vi "hw9p4_hickey.vi"() -> ()   [LabVIEW 2014]
panel:
  out "Prime?":bool
  in  "Integer":dbl
  # "101467 is not prime"
  # "102703 is not prime"
  # "97861 is prime"
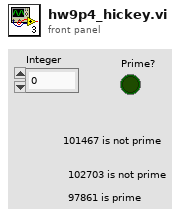
[diagram p1: front panel]
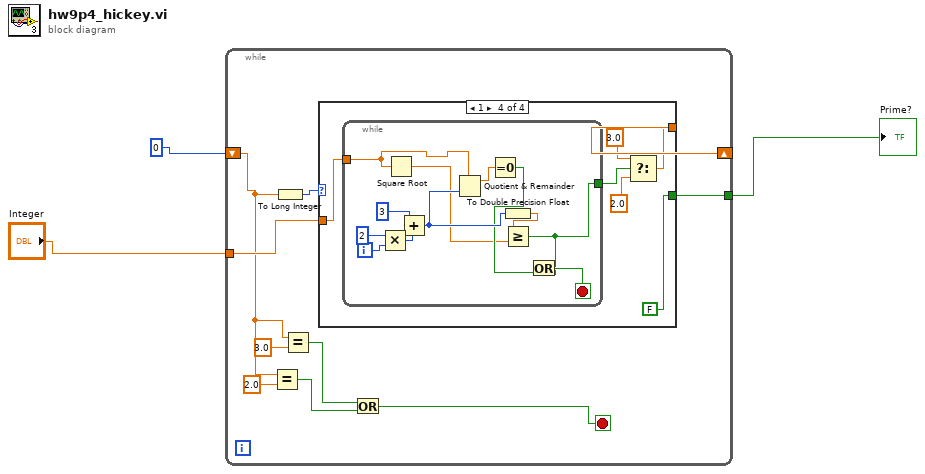
[diagram p0: block diagram]
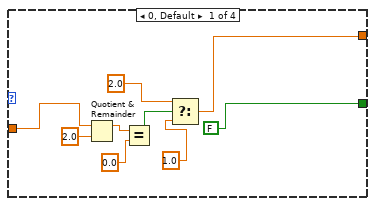
[diagram p2: hidden frame]
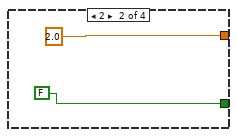
[diagram p3: hidden frame]
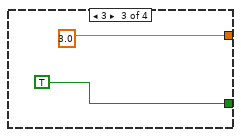
[diagram p4: hidden frame]
diagram:
  n1 = while {
    shift-right: [w12] -> _
    shift-left: 0 -> [w6]
    tunnel: "Integer" -> [w13]
    tunnel: [w4] -> w1
    stop <- w7 stop-if-true
    n2 = Equal?(x=w6, y=2.0) -> (x = y?=w10:bool)
    n3 = To Long Integer(number=w6) -> (32bit integer=w5:i32)
    n4 = Equal?(x=w6, y=3.0) -> (x = y?=w8:bool)
    n5 = case shown="1" w5 {
      tunnel: w13 -> [w21 _ _ w32]
      tunnel: [w15 2.0 ("y") 3.0 ("y") w28] -> w12
      tunnel: [FALSE FALSE TRUE FALSE] -> w4
      frame 0, Default {
        n6 = Quotient & Remainder(x=w21, y=2.0) -> (x-y*floor(x/y)=w19:dbl)  [unwired: 1 out]
        n7 = Equal?(x=w19, y=0.0 ("t")) -> (x = y?=w17:bool)
        n8 = Select(t=2.0, s=w17, f=1.0 ("t")) -> (s? t:f=w15:dbl)
      }
      frame 2 {
      }
      frame 3 {
      }
      frame 1 {
        n9 = while {
          tunnel: w32 -> [w38]
          tunnel: [w33] -> w27
          i -> [w44]
          stop <- w37 stop-if-true
          n10 = Multiply(x=2, y=w44) -> (x*y=w42:i32)
          n11 = Square Root(x=w38) -> (sqrt(x)=w35:dbl)
          n12 = Add(x=3, y=w42) -> (x+y=w39:i32)
          n13 = Quotient & Remainder(x=w38, y=w39) -> (x-y*floor(x/y)=w40:dbl)  [unwired: 1 out]
          n14 = Equal To 0?(x=w40) -> (x = 0?=w36:bool)
          n15 = To Double Precision Float(number=w39) -> (double precision float=w34:dbl)
          n16 = Greater Or Equal?(x=w34, y=w35) -> (x >= y?=w33:bool)
          n17 = Or(x=w33, y=w36) -> (x .or. y?=w37:bool)
        }
        n18 = Select(t=3.0, s=w27, f=2.0 ("t")) -> (s? t:f=w28:dbl)
      }
    }
    n19 = Or(x=w8, y=w10) -> (x .or. y?=w7:bool)
  }
  "Prime?" <- w1
